vi "ROI entry-Previous ROI compat-Frame size.vi"(8 "error in (no error)":errorcluster, 9 "Proceed":bool=TRUE, 11 "Old ROI file path":path) -> (0 "error out":errorcluster, 1 "Proceed":bool, 2 "ROI fit info":T1 {"ROI fit info"."Frame size"."Old" items=["100X100"=100, "128X128"=128, "200X200"=200, "256X256"=256, "512X512"=512, "1024x1024"=1024, "2048x2048"=2048]; "ROI fit info"."Frame size"."New" items=["100X100"=100, "128X128"=128, "200X200"=200, "256X256"=256, "512X512"=512, "1024x1024"=1024, "2048x2048"=2048]}, 3 "Old ROI file path (dup)":path)   [LabVIEW 2013]
uses:
  Typedefs/ROI fitting info cluster.ctl
  Typedefs/Frame Size.ctl
  Visualisation/Functional Imaging Viewer/SubVIs/Experiment header interface/Typedefs/Header file type enum.ctl
  Visualisation/Functional Imaging Viewer/SubVIs/Experiment header interface/Typedefs/Save-Load-Save as-Load last enum.ctl
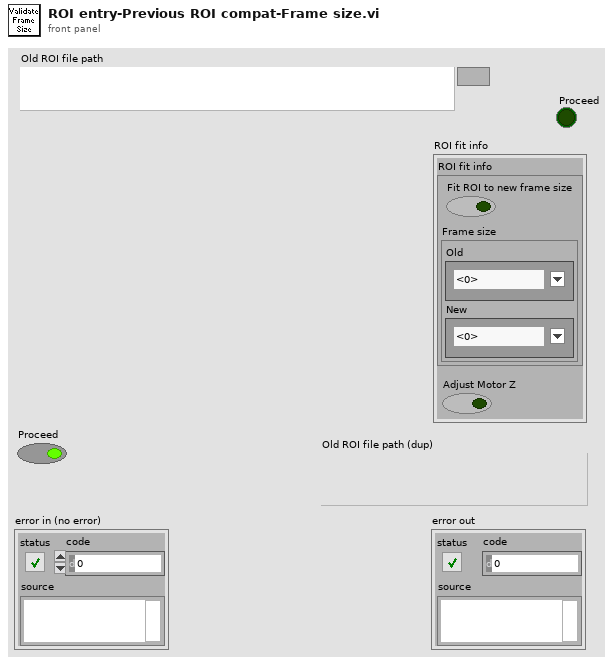
[diagram p1: front panel]
types:
  T1 = typedef "ROI fitting info cluster.ctl" = cluster{"ROI fit info":cluster{"Fit ROI to new frame size":bool, "Frame size":cluster{"Old":T2, "New":T2}}, "Adjust Motor Z":bool}
  T2 = typedef "Frame Size.ctl" = u16
  T3 = typedef "Save-Load-Save as-Load last enum.ctl" = enum16{"Save file", "Save file as", "Load file", "Load last file"}
  T4 = typedef "Header file type enum.ctl" = enum16{"All parameters", "Params for funct acq w ROI or mscn", "Params for funct acq w rectangles", "Live imaging header parameters", "AOL Parameters"}
  T5 = typedef "Fixed strings.ctl" = cluster{"ROI file name":string, "Normalised ROI file name":string, "Zplane Pockels values file name":string, "Functional data folder name":string, "Experiment Header file name":string, "Z-stack images folder name":string, "Groups setup rel. path":string, "Groups text file rel. path":string, "TDMS files folder name (F.img)":string, "TDMS files folder name (V.acq)":string, "TDMS files folder name (Pl.acq)":string, "Cycle rel times sequence file":string, "Dynamically called VIs folder name":string, "Time Series folder base name":string}
  T6 = typedef "Header parameters cluster-ALL.ctl" = cluster{"Imaging Protocol":T7, "Number of POI":u16, "Number of Miniscans":u16, "Number of Trials":u16, "Number of Cycles ":u64, "# Averaged Frames":u16, "Laser power (%)":u8, "Pockels":dbl, "Acquisition Length (sec)":dbl, "Fill time (us)":dbl, "POI Dwell time (us)":dbl, "Miniscan Dwell time per pixel (us)":dbl, "PMT 1":dbl, "PMT 2":dbl, "Back Apperture":dbl, "Zoom":dbl, "Frame Size":T2, "Center Frequency":dbl, "Field of View":dbl, "DwellTime (us)":dbl, "Wavelength (nm)":dbl, "AOL Z":dbl, "AOL Mode":T8, "GridXY":dbl, "GridZ":dbl, "TriggerDelay (sec)":dbl, "Number of Pixels in Miniscan":u16, "Experiment folder path":path, "X centre":dbl, "Y centre":dbl, "Angle (degrees)":dbl, "Plane Mode":T9, "Software version":dbl, "Objective":T10, "MotorZ Calibration":u32, "Pockels Calibration":u32, "Threshold":u16[], "Video length (sec)":dbl, "Frame rate (fps)":u8, "Rectangle ROI length (pixels)":u16, "Rectangle ROI height (pixels)":u16}
  T7 = typedef "Imaging Protocols enum.ctl" = enum16{"AOL Z-Stack", "Motor Z Stack", "Functional Acquisition", "Single Plane Acquisition", "Volume Acquisition", "Live Imaging", "Live Plane Imaging", "Live Volume Imaging"}
  T8 = typedef "AOL modes.ctl" = enum16{"Raster", "Structural", "Pointing", "Mini Scan", "Alignment"}
  T9 = typedef "Plane Mode.ctl" = u16
  T10 = typedef "Objective selector control enum.ctl" = string
  T11 = typedef "AOL_Globals.ctl" = cluster{"Imaging Protocol":T7, "Number of POI":u16, "Number of Miniscans":u16, "Number of Trials":u16, "Number of Cycles ":u64, "# Averaged Frames":u16, "Laser power (%)":u8, "Pockels":dbl, "Acquisition Length (sec)":dbl, "Fill time (us)":dbl, "POI Dwell time (us)":dbl, "Miniscan Dwell time per pixel (us)":dbl, "PMT 1":dbl, "PMT 2":dbl, "Back Apperture":dbl, "Frame Size":T2, "Center Frequency":dbl, "Field of View":dbl, "DwellTime (us)":dbl, "Wavelength (nm)":dbl, "Zoom":dbl, "AOL Z":dbl, "AOL Mode":T8, "GridXY":dbl, "GridZ":dbl, "TriggerPeriod (sec)":dbl, "Number of Pixels in Miniscan":u16, "Experiment folder path":path, "X centre":dbl, "Y centre":dbl, "Angle (degrees)":dbl, "Plane Mode":T9, "Threshold":u16[], "Regenerate Chirps":bool, "Rectangle ROI length (pixels)":u16, "Rectangle ROI height (pixels)":u16, "AOD fill":u16, "Samples Wait after Trigger":u16, "StartUp Delay":i32, "Slip Cycle":u32, "Add Cycle":bool}
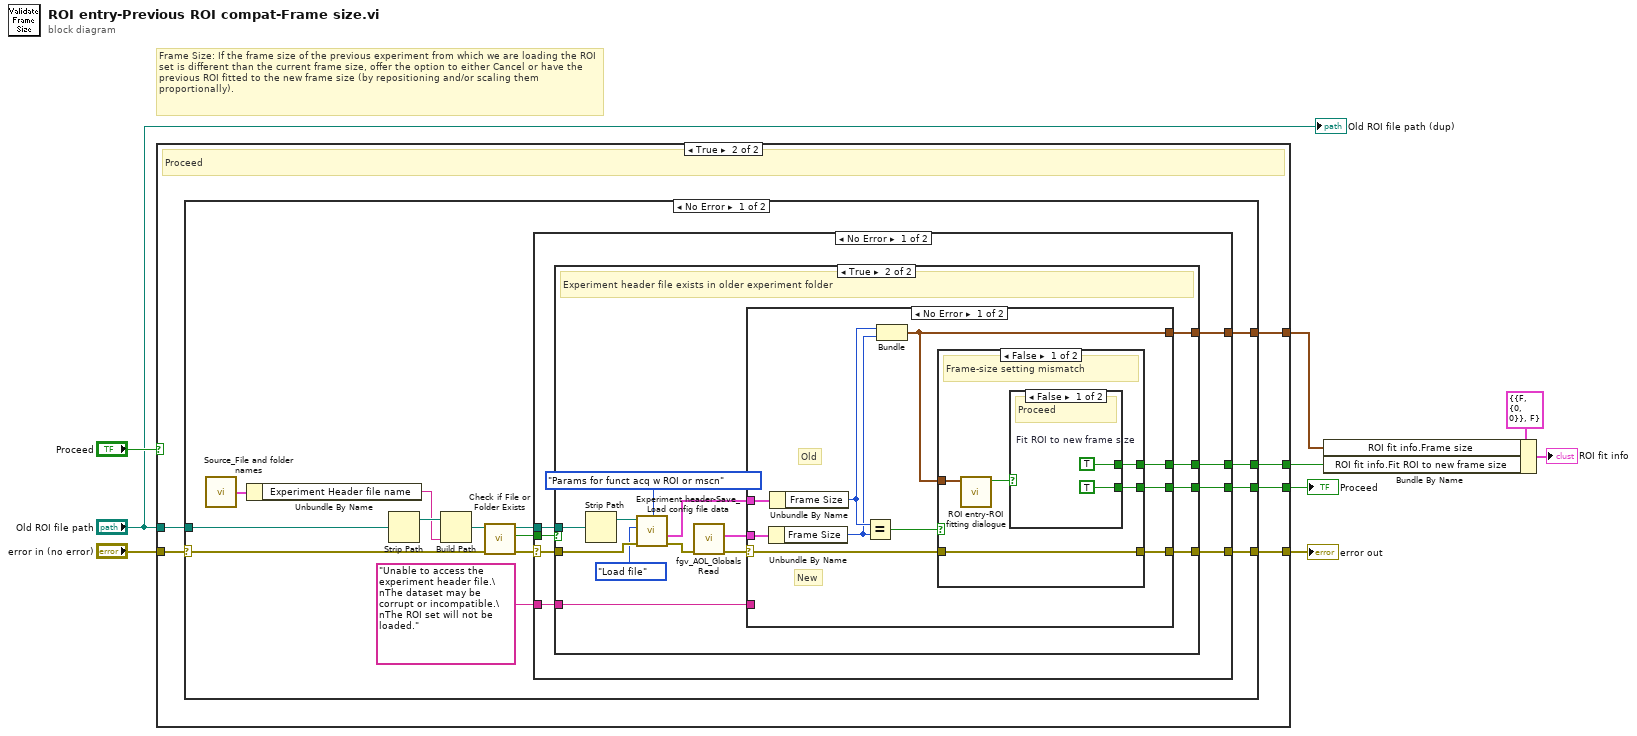
[diagram p0: block diagram]
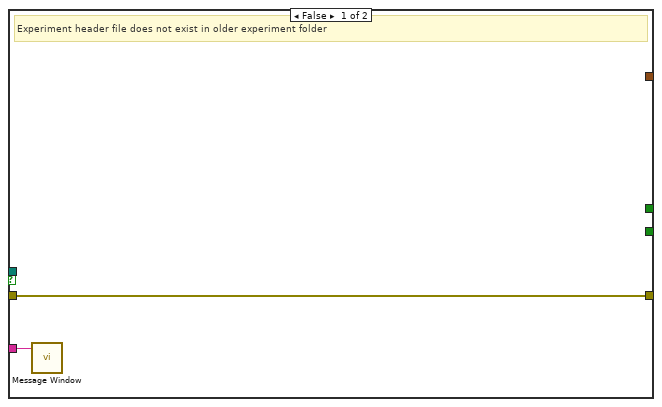
[diagram p3: hidden frame]
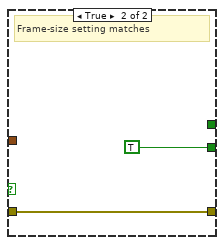
[diagram p5: hidden frame]
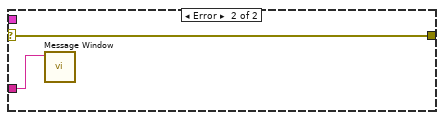
[diagram p6: hidden frame]
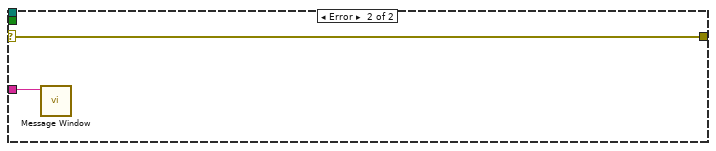
[diagram p7: hidden frame]
diagram:
  # "Frame Size: If the frame size of the previous experiment from which we are loading the ROI set is different than the current frame size, offer the option to either Cancel or have the previous ROI fitted to the new frame size (by repositioning and/or scaling them proportionally)."
  n1 = case shown="True" "Proceed" {
    tunnel: "Old ROI file path" -> [_ w16]
    tunnel: [w10 w15] -> w9
    tunnel: "error in (no error)" -> [w10 w14]
    tunnel: [_ w13] -> w7
    tunnel: [_ w12] -> w4
    tunnel: [_ w11] -> w1
    frame False {
      # "Skip"
    }
    frame True {
      # "Proceed"
      n2 = case shown="No Error" w14 {
        selector: w14 -> [w21 w78]
        tunnel: w16 -> [w28 _]
        tunnel: [w24 _] -> w13
        tunnel: [w20 w78] -> w15
        tunnel: [w18 _] -> w12
        tunnel: [w17 _] -> w11
        frame No Error {
          n3 = call "Source_File and folder names.vi"() -> ("Fixed strings"=w29:T5)  [unwired: 1 in]
          n4 = Unbundle By Name(w29) -> ("Experiment Header file name"=w26:string)
          n5 = Strip Path(path=w28) -> (stripped path=w27:path)  [unwired: 1 out]
          n6 = Build Path(base path=w27, name or relative path=w26) -> (appended path=w30:path)
          n7 = call <vilib>:"Check if File or Folder Exists.vi"("error in (no error)"=w21, "path"=w30) -> ("error out"=w22:errorcluster, "file or folder exists?"=w25:bool, "dup path"=w23:path)  [unwired: 7 in]
          n8 = case shown="No Error" w22 {
            selector: w22 -> [w35 w77]
            tunnel: w25 -> [w38 _]
            tunnel: [w37 _] -> w24
            tunnel: w23 -> [w36 _]
            tunnel: [w34 w77] -> w20
            tunnel: "Unable to access the experiment header file.\nThe dataset may be corrupt or incompatible.\nThe ROI set will not be loaded." ("Message string") -> [w33 w76]
            tunnel: [w32 _] -> w18
            tunnel: [w31 _] -> w17
            frame No Error {
              n9 = case shown="True" w38 {
                tunnel: [_ w48] -> w37
                tunnel: w36 -> [_ w52]
                tunnel: w35 -> [w40 w50]
                tunnel: [w40 w47] -> w34
                tunnel: w33 -> [w39 w43]
                tunnel: [_ w42] -> w32
                tunnel: [_ w41] -> w31
                frame False {
                  # "Experiment header file does not exist in older experiment folder"
                  n10 = call "Message Window.vi"("Message string"=w39) -> ()  [unwired: 10 in, 1 out]
                }
                frame True {
                  # "Experiment header file exists in older experiment folder"
                  n11 = Strip Path(path=w52) -> (stripped path=w51:path)  [unwired: 1 out]
                  n12 = call "Experiment header-Save_Load config file data.vi"("Header file type"=Header_file_type_enum."Params for funct acq w ROI or mscn", "error in (no error)"=w50, "Function"=Save-Load-Save_as-Load_last_enum."Load file", "Experiment data folder path"=w51) -> ("error out"=w49:errorcluster, "All header parameters out"=w53:T6)  [unwired: 6 in]
                  n13 = call "fgv_AOL_Globals Read.vi"("error in (no error)"=w49) -> ("error out"=w46:errorcluster, "AOL_Globals"=w54:T11)  [unwired: 8 in, 1 out]
                  n14 = case shown="No Error" w46 {
                    selector: w46 -> [w60 w75]
                    tunnel: w54 -> [w59 _]
                    tunnel: w53 -> [w64 _]
                    tunnel: [w62 _] -> w48
                    tunnel: [w61 w75] -> w47
                    tunnel: w43 -> [_ w74]
                    tunnel: [w58 _] -> w42
                    tunnel: [w55 _] -> w41
                    frame No Error {
                      # "New"
                      # "Old"
                      n15 = Unbundle By Name(w59) -> ("Frame Size"=w56:T2)
                      n16 = Unbundle By Name(w64) -> ("Frame Size"=w57:T2)
                      n17 = Equal?(x=w57, y=w56) -> (x = y?=w63:bool)
                      n18 = Bundle("Frame Size"=w57, "Frame Size"=w56) -> (w55:cluster{"Frame Size":T2, "Frame Size":T2})  [unwired: 1 in]
                      n19 = case shown="False" w63 {
                        tunnel: [w68 TRUE] -> w62
                        tunnel: w60 -> [w67 w72]
                        tunnel: [w67 w72] -> w61
                        tunnel: [w66 _] -> w58
                        tunnel: w55 -> [w65 _]
                        frame False {
                          # "Frame-size setting mismatch"
                          n20 = call "ROI entry-ROI fitting dialogue.vi"("Frame size"=w65) -> ("Cancelled (Left button pressed)"=w69:bool)  [unwired: 10 in]
                          n21 = case shown="False" w69 {
                            tunnel: [TRUE _] -> w68
                            tunnel: [w70 _] -> w66
                            frame False {
                              w70 = TRUE  # Fit ROI to new frame size
                              # "Proceed"
                            }
                            frame True {
                              # "Cancelled"
                            }
                          }
                        }
                        frame True {
                          # "Frame-size setting matches"
                        }
                      }
                    }
                    frame Error {
                      n22 = call "Message Window.vi"("Message string"=w74) -> ()  [unwired: 10 in, 1 out]
                    }
                  }
                }
              }
            }
            frame Error {
              n23 = call "Message Window.vi"("Message string"=w76) -> ()  [unwired: 10 in, 1 out]
            }
          }
        }
        frame Error {
        }
      }
    }
  }
  "error out" <- w9
  "Proceed" <- w7
  n24 = Bundle By Name(cluster=T1 {"ROI fit info"={"Fit ROI to new frame size"=FALSE, "Frame size"={"Old"=0, "New"=0}}, "Adjust Motor Z"=FALSE} ("ROI fit info"), "ROI fit info.Frame size"=w1, "ROI fit info.Fit ROI to new frame size"=w4) -> (→"ROI fit info":T1)
  "Old ROI file path (dup)" <- "Old ROI file path"
